vi "comms_BT_Read_TXT.vi"(8 "error in":errorcluster, 10 "timeout ms (25000)":i32, 11 "connection ID":refnum<k31>) -> (0 "error out":errorcluster, 1 "Read Count":i32, 2 "Data Out":string, 3 "connection ID Out":refnum<k31>)   [LabVIEW 2018]
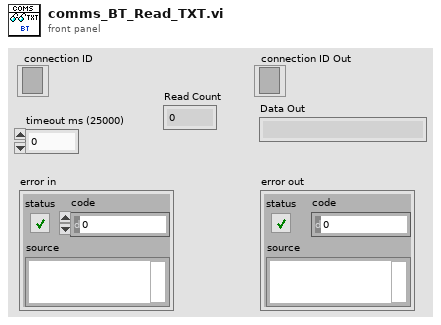
[diagram p1: front panel]
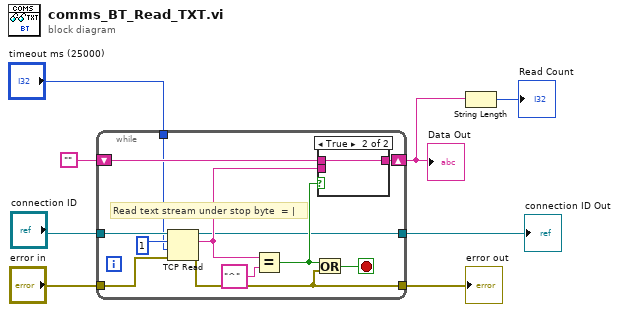
[diagram p0: block diagram]
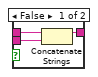
[diagram p2: hidden frame]
diagram:
  n1 = while {
    tunnel: [w12] -> w7
    tunnel: "error in" -> [w14]
    shift-right: [w17] -> w6
    shift-left: "" -> [w18]
    tunnel: "connection ID" -> [w15]
    tunnel: [w10] -> w2
    tunnel: "timeout ms (25000)" -> [w9]
    stop <- w20 stop-if-true
    # "Read text stream under stop byte  = |"
    n2 = TCP Read(connection ID=w15, bytes to read=u32 1 ("byte count"), error in (no error)=w14, 9:w9) -> (connection ID out=w10:refnum<k31>, data out=w11:string, error out=w12:errorcluster)  [unwired: 1 in]
    n3 = Equal?(x=w11, y="^") -> (x = y?=w16:bool)
    n4 = Or(x=w16, y=w12) -> (x .or. y?=w20:bool)
    n5 = case shown="True" w16 {
      tunnel: w18 -> [w23 w24]
      tunnel: w11 -> [w22 _]
      tunnel: [w21 w24] -> w17
      frame False {
        n6 = Concatenate Strings(w23, w22) -> (w21:string)
      }
      frame True {
      }
    }
  }
  "error out" <- w7
  "Data Out" <- w6
  "connection ID Out" <- w2
  n7 = String Length(string=w6) -> (length=→"Read Count":i32)
